vi "applyNewDelays.vi"(8 "error in (no error)":errorcluster, 11 "ScriptEventList in":refnum<class "ScriptEventList.lvclass">) -> (0 "error out":errorcluster, 3 "ScriptEventList out":refnum<class "ScriptEventList.lvclass">)   [LabVIEW 2011, in "Tools.lvlib" / "Scripting.lvlib" / "ScriptEventList.lvclass"]
uses:
  ScriptEventList.lvclass
  ScriptEventList.lvclass/ScriptEventList.ctl
  ScriptEvent.lvclass
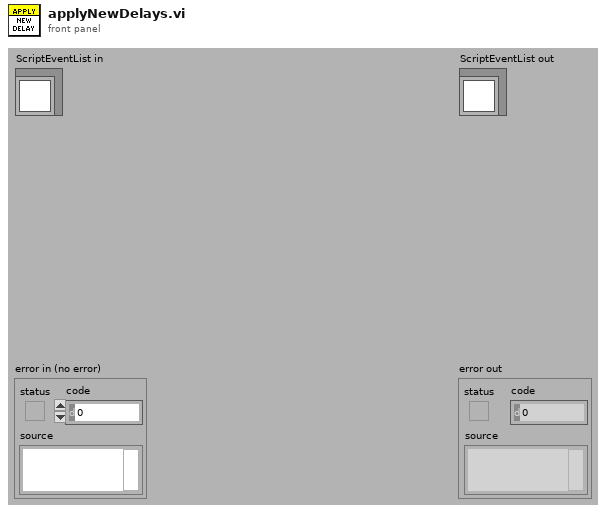
[diagram p1: front panel]
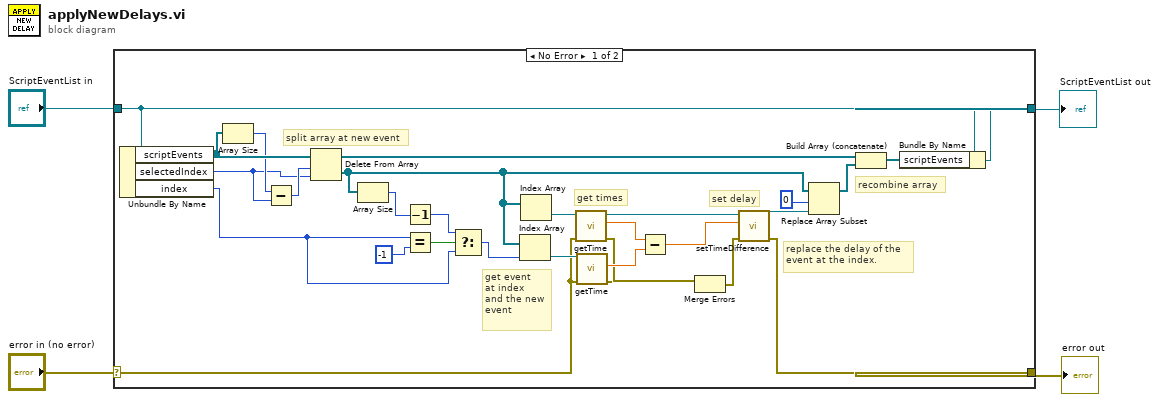
[diagram p0: block diagram]
diagram:
  n1 = case shown="No Error" "error in (no error)" {
    selector: "error in (no error)" -> [w22 w35]
    tunnel: [w6 w35] -> w3
    tunnel: [w7 w34] -> w1
    tunnel: "ScriptEventList in" -> [w8 w34]
    frame No Error {
      # "replace the delay of the \nevent at the index."
      # "get event\nat index\nand the new\nevent"
      # "split array at new event"
      # "recombine array"
      # "set delay"
      # "get times"
      n2 = Unbundle By Name(w8) -> ("scriptEvents"=w33:refnum<class "ScriptEvent.lvclass">[], "selectedIndex"=w5:i32, "index"=w26:i32)
      n3 = Array Size(array=w33) -> (size(s)=w32:i32)
      n4 = Subtract(x=w32, y=w5) -> (x-y=w31:i32)
      n5 = Delete From Array(array=w33, length=w31, index=w5) -> (deleted portion=w14:refnum<class "ScriptEvent.lvclass">[], array with subset deleted=w11:refnum<class "ScriptEvent.lvclass">[])
      n6 = Array Size(array=w14) -> (size(s)=w28:i32)
      n7 = Decrement(x=w28) -> (x-1=w27:i32)
      n8 = Equal?(x=w26, y=-1) -> (x = y?=w30:bool)
      n9 = Select(t=w27, s=w30, f=w26) -> (s? t:f=w25:i32)
      n10 = Index Array(array=w14, index=w25) -> (element=w24:refnum<class "ScriptEvent.lvclass">)
      n11 = Index Array(array=w14) -> (element=w23:refnum<class "ScriptEvent.lvclass">)  [unwired: 1 in]
      n12 = call "getTime.vi"("error in (no error)"=w22, "ScriptEvent.lvclass in"=w23) -> ("error out"=w17:errorcluster, "time"=w21:dbl, "ScriptEvent.lvclass out"=w19:refnum<class "ScriptEvent.lvclass">)  [unwired: 7 in]
      n13 = call "getTime.vi"("error in (no error)"=w22, "ScriptEvent.lvclass in"=w24) -> ("error out"=w16:errorcluster, "time"=w20:dbl)  [unwired: 7 in, 1 out]
      n14 = Subtract(x=w21, y=w20) -> (x-y=w18:dbl)
      n15 = Merge Errors(w17, w16) -> (w15:errorcluster)
      n16 = call "setTimeDifference.vi"("error in (no error)"=w15, "time difference"=w18, "ScriptEvent.lvclass in"=w19) -> ("error out"=w6:errorcluster, "ScriptEvent.lvclass out"=w13:refnum<class "ScriptEvent.lvclass">)  [unwired: 7 in]
      n17 = Replace Array Subset(array=w14, new element=w13, index=0) -> (w10:refnum<class "ScriptEvent.lvclass">[])
      n18 = Build Array (concatenate)(w11, w10) -> (w9:refnum<class "ScriptEvent.lvclass">[])
      n19 = Bundle By Name(cluster=w8, "scriptEvents"=w9) -> (w7:refnum<class "ScriptEventList.lvclass">)
    }
    frame Error {
    }
  }
  "error out" <- w3
  "ScriptEventList out" <- w1
